vi "Read constants.vi"(9 "Diagram in":refnum<class "Diagram.lvclass">) -> (3 "Diagram out":refnum<class "Diagram.lvclass">, 4 "constants":refnum<class "Constant.lvclass">[](array[class]))   [LabVIEW 2014, in "Raspberry Pi Compatible Compiler for LabVIEW.lvlib" / "Diagram.lvclass"]
uses:
  Diagram.lvclass
  Constant/Constant.lvclass
  Diagram.lvclass/Diagram.ctl
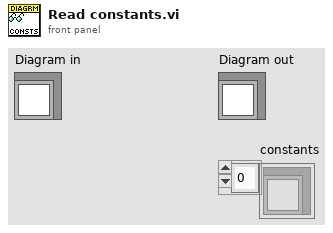
[diagram p1: front panel]
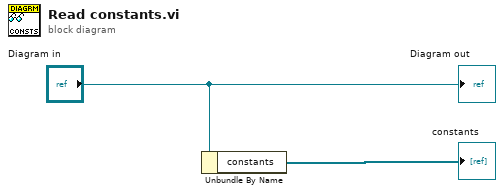
[diagram p0: block diagram]
diagram:
  n1 = Unbundle By Name("Diagram in") -> ("constants"=→"constants":refnum<class "Constant.lvclass">[])
  "Diagram out" <- "Diagram in"
